vi "Destroy.vi"(8 "Error In":errorcluster, 11 "object in":refnum<class "Component.lvclass">) -> (0 "Error Out":errorcluster)   [LabVIEW 2020, in "Component.lvclass"]
uses:
  Component.lvclass
  Component.lvclass/Component.ctl
  <vilib>/sklein/WebView2/Webview2 Lib/WebView2 Control Object/WebView2 Control.lvclass
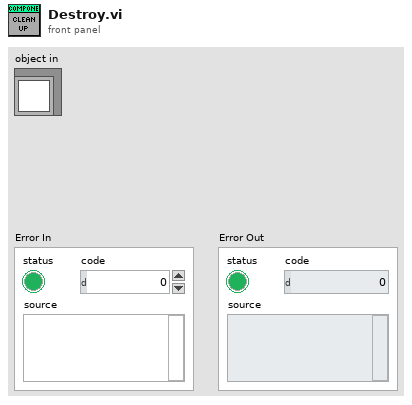
[diagram p1: front panel]
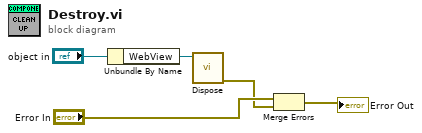
[diagram p0: block diagram]
diagram:
  n1 = Unbundle By Name("object in") -> ("WebView"=w2:refnum<class "WebView2 Control.lvclass">)
  n2 = call <vilib>:"Dispose.vi"("WebView2 Control in"=w2) -> ("error out"=w1:errorcluster)  [unwired: 10 in]
  n3 = Merge Errors("Error In", w1) -> (→"Error Out":errorcluster)
